vi "TTRM Analyze Thermistor ABC Parameters.vi"(0 "Thermistor Parameters":T2 {"Beta Parameters"."R0 (Ohm)" format="%#.6p"; "Beta Parameters"."Beta Value (K)" format="%#.6p"; "ABC Parameters"."C" format="%^.6e"; "ABC Parameters"."B" format="%^.6e"; "ABC Parameters"."A" format="%^.6e"}, 11 "error in (no error)":errorcluster) -> (4 "ABC Parameters":T1 {"C" format="%^.6e"; "B" format="%^.6e"; "A" format="%^.6e"}, 15 "error out":errorcluster)   [LabVIEW 2021, in "DAQ_Temperature Thermistor Measurement.lvlib"]
doc: "Gets the thermistor parameters as input and derives the <B>Steinhart–Hart A B C</B> parameters which are used to obtain Temperature measurements."
uses:
  DAQ_Temperature Thermistor Measurement.lvlib
  Typedefs/ABC Parameters.ctl
  Typedefs/Beta Parameters.ctl
  Typedefs/Thermistor Parameters.ctl
panel:
  # "Inputs"
  # "Outputs"
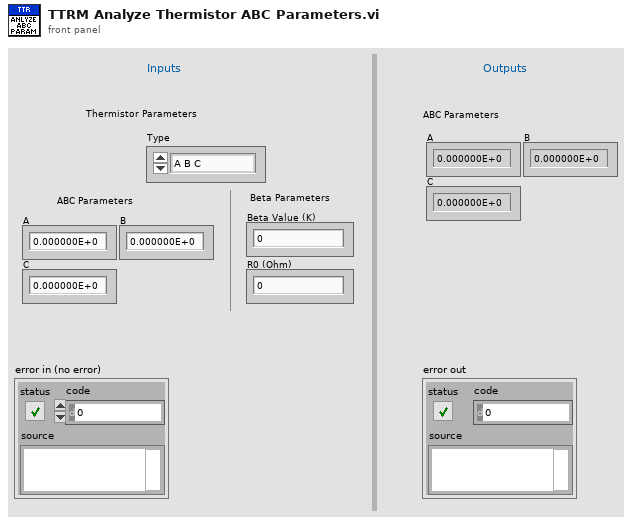
[diagram p1: front panel]
types:
  T1 = typedef "DAQ_Temperature Thermistor Measurement.lvlib/ABC Parameters.ctl" = cluster{"A":dbl, "B":dbl, "C":dbl}
  T2 = typedef "DAQ_Temperature Thermistor Measurement.lvlib/Thermistor Parameters.ctl" = cluster{"Type":enum16{"A B C", "Beta"}, "ABC Parameters":T1, "Beta Parameters":T3}
  T3 = typedef "DAQ_Temperature Thermistor Measurement.lvlib/Beta Parameters.ctl" = cluster{"Beta Value (K)":dbl, "R0 (Ohm)":dbl}
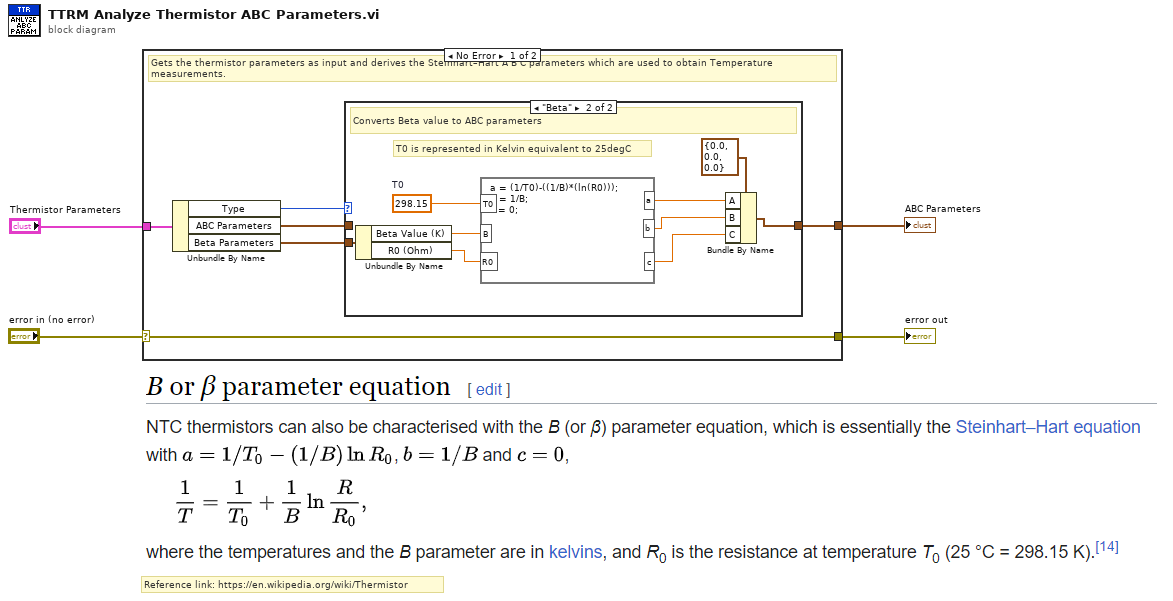
[diagram p0: block diagram]
diagram:
  # "Reference link: https://en.wikipedia.org/wiki/Thermistor"
  n1 = case shown="No Error" "error in (no error)" {
    selector: "error in (no error)" -> [w10 w21]
    tunnel: [w10 w21] -> w3
    tunnel: "Thermistor Parameters" -> [w9 _]
    tunnel: [w6 _] -> w1
    frame No Error {
      # "Gets the thermistor parameters as input and derives the Steinhart–Hart A B C parameters which are used to obtain Temperature measurements."
      n2 = Unbundle By Name(w9) -> ("Type"=w8:enum16{"A B C", "Beta"}, "ABC Parameters"=w7:T1, "Beta Parameters"=w5:T3)
      n3 = case shown="\"Beta\"" w8 {
        tunnel: w7 -> [w11 _]
        tunnel: [w11 w12] -> w6
        tunnel: w5 -> [_ w20]
        frame "A B C", Default {
          # "ABC value is taken as default"
        }
        frame "Beta" {
          w18 = 298.15  # T0
          # "T0 is represented in Kelvin equivalent to 25degC"
          # "Converts Beta value to ABC parameters"
          n4 = Unbundle By Name(w20) -> ("Beta Value (K)"=w17:dbl, "R0 (Ohm)"=w16:dbl)
          n5 = formula code="a = (1/T0)-((1/B)*(ln(R0)));\nb = 1/B;\nc = 0;"("T0"=w18, "B"=w17, "R0"=w16) -> ("a"=w15:dbl, "b"=w14:dbl, "c"=w13:dbl)
          n6 = Bundle By Name(cluster=T1 {"A"=0.0, "B"=0.0, "C"=0.0} ("ABC Parameters"), "A"=w15, "B"=w14, "C"=w13) -> (w12:T1)
        }
      }
    }
    frame Error {
      # "Error case - Do nothing"
    }
  }
  "ABC Parameters" <- w1
  "error out" <- w3
